vi "squiggle_init.vi"(8 "Error in":errorcluster, 11 "I2C interface":T1) -> (0 "Error out":errorcluster)   [LabVIEW 2013]
uses:
  i2c_interface.ctl
  fpga_reference.ctl
panel:
  # "Start the I2C interface on the FPGA target and send the calibration initialization sequences to the motor drivers.  This takes approximately 200 ms."
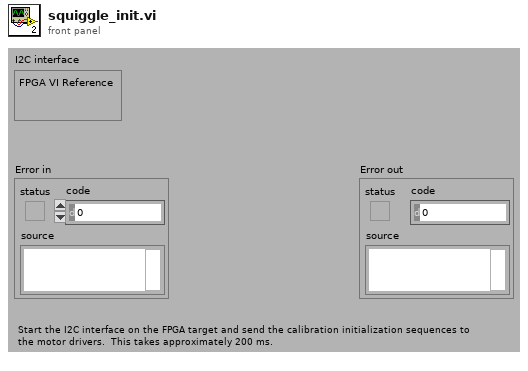
[diagram p1: front panel]
types:
  T1 = typedef "i2c_interface.ctl" = cluster{"FPGA VI Reference":T2}
  T2 = typedef "fpga_reference.ctl" = refnum<k20>
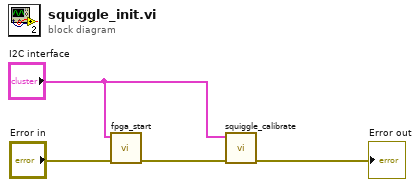
[diagram p0: block diagram]
diagram:
  n1 = call "fpga_start.vi"("error in"="Error in", "I2C interface"="I2C interface") -> ("error out"=w3:errorcluster)  [unwired: 9 in]
  n2 = call "squiggle_calibrate.vi"("error in"=w3, "I2C interface"="I2C interface") -> ("error out"=→"Error out":errorcluster)  [unwired: 9 in]
